vi "Read Chart Scales.vi"(8 "error in (no error)":errorcluster, 11 "Chart in":refnum<vi>) -> (0 "error out":errorcluster, 2 "Chart Scales":T1, 3 "Chart":refnum<vi>)   [LabVIEW 2020, in "VolatusGUIEditorCore.lvlib"]
uses:
  VolatusGUIEditorCore.lvlib
  Chart Scale Props.ctl
  Chart Scales.ctl
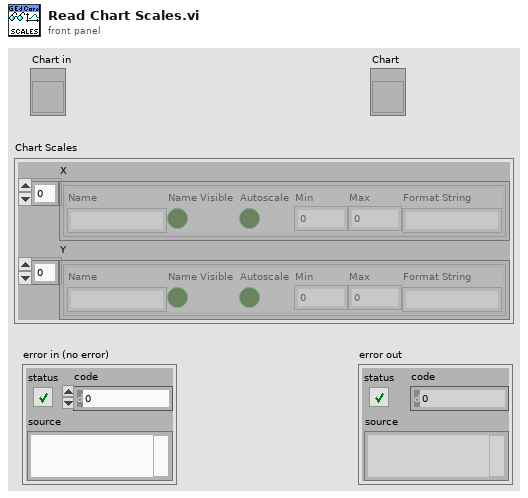
[diagram p1: front panel]
types:
  T1 = typedef "VolatusGUIEditorCore.lvlib/Chart Scales.ctl" = cluster{"X":T2[], "Y":T2[]}
  T2 = typedef "VolatusGUIEditorCore.lvlib/Chart Scale Props.ctl" = cluster{"Name":string, "Name Visible":bool, "Autoscale":bool, "Min":dbl, "Max":dbl, "Format String":string}
  T3 = typedef "VolatusGUIEditorCore.lvlib/Chart Scale Count.ctl" = cluster{"X":i32, "Y":i32}
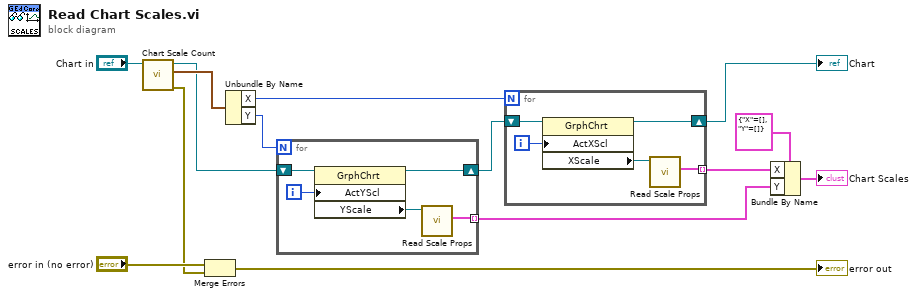
[diagram p0: block diagram]
diagram:
  n1 = call "Chart Scale Count.vi"("Chart in"="Chart in") -> ("error out"=w1:errorcluster, "Chart Scale Count"=w13:T3, "Chart"=w5:refnum<vi>)  [unwired: 8 in]
  n2 = Merge Errors("error in (no error)", w1) -> (→"error out":errorcluster)
  n3 = Unbundle By Name(w13) -> ("X"=w11:i32, "Y"=w12:i32)
  n4 = for {
    N: w12 -> [_]
    tunnel: [w16] -> w6 mode=indexing
    shift-right: [w15] -> w10
    shift-left: w5 -> [w19]
    i -> [w18]
    n5 = property class="GrphChrt"(reference=w19, "ActYScl"=w18) -> (reference out=w15:refnum<vi>, "YScale"=w17:refnum<vi>)  [unwired: 1 in, 1 out]
    n6 = call "Read Scale Props.vi"("GraphScale"=w17) -> ("GraphScale Props"=w16:T2)  [unwired: 10 in]
  }
  n7 = for {
    N: w11 -> [_]
    tunnel: [w21] -> w7 mode=indexing
    shift-right: [w20] -> w4
    shift-left: w10 -> [w24]
    i -> [w23]
    n8 = property class="GrphChrt"(reference=w24, "ActXScl"=w23) -> (reference out=w20:refnum<vi>, "XScale"=w22:refnum<vi>)  [unwired: 1 in, 1 out]
    n9 = call "Read Scale Props.vi"("GraphScale"=w22) -> ("GraphScale Props"=w21:T2)  [unwired: 10 in]
  }
  "Chart" <- w4
  n10 = Bundle By Name(cluster=T1 {"X"=[], "Y"=[]} ("Chart Scales"), "X"=w7, "Y"=w6) -> (→"Chart Scales":T1)
